vi "Global 3.vi"() -> ()   [LabVIEW 2015]
panel:
  in  "Numeric 2":dbl
  in  "Numeric":dbl
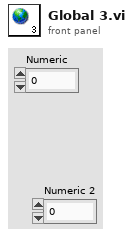
[diagram p1: front panel]
diagram:
